vi "equals.vi"(8 "error in (no error)":errorcluster, 10 "object 2":refnum<class>, 11 "pRectangle in":refnum<class "pRectangle.lvclass">) -> (0 "error out":errorcluster, 2 "equal?":bool, 3 "pRectangle out":refnum<class "pRectangle.lvclass">)   [LabVIEW 2017, in "pRectangle.lvclass"]
uses:
  pRectangle.lvclass
  pRectangle.lvclass/pRectangle.ctl
  Shape Class/pShape.lvclass
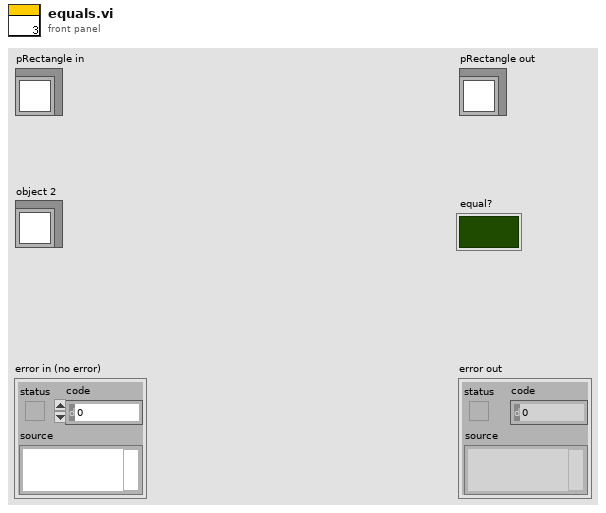
[diagram p1: front panel]
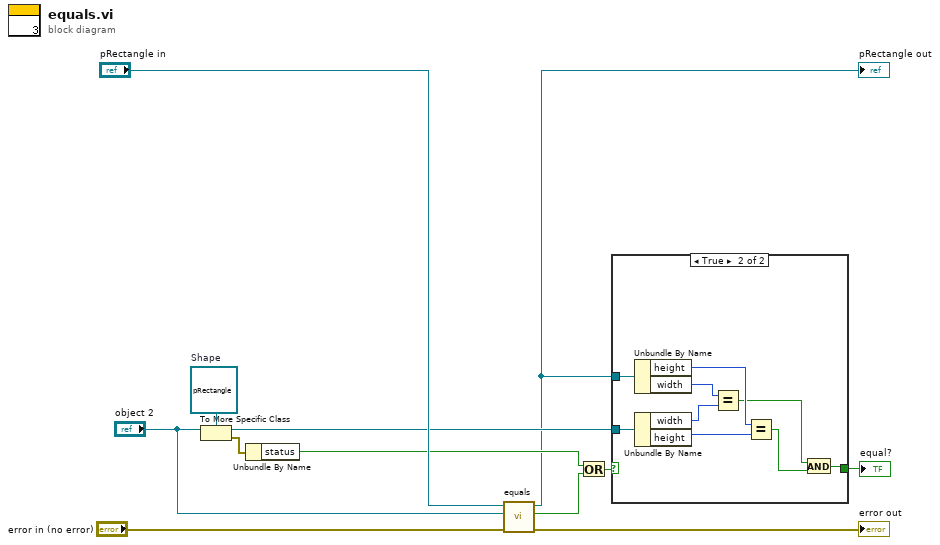
[diagram p0: block diagram]
diagram:
  w8 = refnum<class "pRectangle.lvclass"> refnum  # Shape
  n1 = To More Specific Class(target class=w8, reference="object 2") -> (specific class reference=w2:refnum<class "pRectangle.lvclass">, error out=w9:errorcluster)  [unwired: 1 in]
  n2 = Unbundle By Name(w9) -> ("status"=w5:bool)
  n3 = call-parent "equals.vi"("error in (no error)"="error in (no error)", "object 2"="object 2", "pShape in"="pRectangle in") -> ("error out"=→"error out":errorcluster, "equal?"=w6:bool, "pShape out"=w1:refnum<class "pRectangle.lvclass">)  [unwired: 6 in]
  "pRectangle out" <- w1
  n4 = Or(x=w5, y=w6) -> (x .or. y?=w4:bool)
  n5 = case shown="True" w4 {
    selector: w4 -> [w13 _]
    tunnel: [w13 w16] -> w3
    tunnel: w2 -> [_ w21]
    tunnel: w1 -> [_ w22]
    frame False {
    }
    frame True {
      n6 = Unbundle By Name(w22) -> ("height"=w18:i32, "width"=w20:i32)
      n7 = Unbundle By Name(w21) -> ("width"=w19:i32, "height"=w17:i32)
      n8 = Equal?(x=w20, y=w19) -> (x = y?=w15:bool)
      n9 = Equal?(x=w18, y=w17) -> (x = y?=w14:bool)
      n10 = And(x=w15, y=w14) -> (x .and. y?=w16:bool)
    }
  }
  "equal?" <- w3
